vi "unpackAutonArray.vi"(9 "all rows":dbl[][](array[numeric])) -> (0 "Power":dbl[](array[numeric]), 1 "Distance/Time":dbl[](array[numeric]), 2 "Heading":dbl[](array[numeric]), 3 "Primitive":i16[](array[numeric]), 4 "Misc":dbl[](array[numeric]))   [LabVIEW 2012]
doc: "Use this VI to separate the autonomous array data into individual arrays. First array is Primitive ID, second is heading, etc."
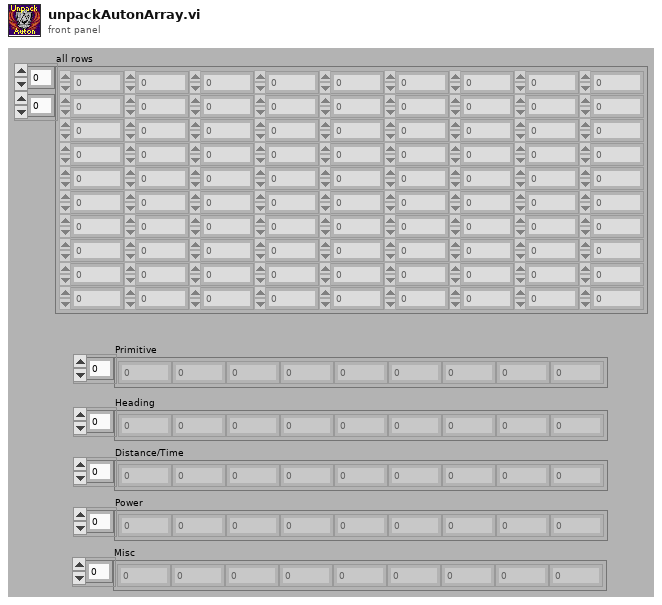
[diagram p1: front panel]
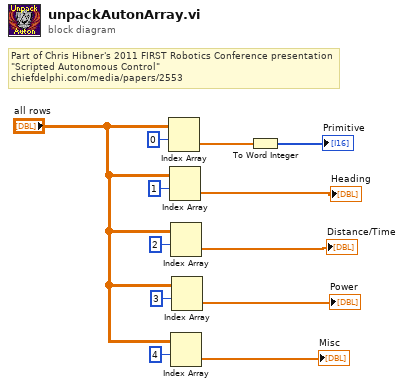
[diagram p0: block diagram]
diagram:
  # "Part of Chris Hibner's 2011 FIRST Robotics Conference presentation\n\"Scripted Autonomous Control\"\nchiefdelphi.com/media/papers/2553"
  n1 = Index Array(array="all rows", index (row)=0) -> (element=w7:dbl[])  [unwired: 1 in]
  n2 = Index Array(array="all rows", index (row)=1) -> (element=→"Heading":dbl[])  [unwired: 1 in]
  n3 = Index Array(array="all rows", index (row)=2) -> (element=→"Distance/Time":dbl[])  [unwired: 1 in]
  n4 = Index Array(array="all rows", index (row)=4) -> (element=→"Misc":dbl[])  [unwired: 1 in]
  n5 = Index Array(array="all rows", index (row)=3) -> (element=→"Power":dbl[])  [unwired: 1 in]
  n6 = To Word Integer(number=w7) -> (16bit integer=→"Primitive":i16[])
